vi "DAQ_2.vi"() -> ()   [LabVIEW 2021]
panel:
  in  "Fase":dbl(knob) scale=0.0..180.0
  in  "Frecuencia":dbl(knob) scale=0.0..30.0
  in  "Offset":dbl(knob) scale=-5.0..5.0
  in  "Amplitud":dbl(knob) scale=-5.0..5.0
  in  "Stop":bool
  out "Sine":dynamicdata(graph)
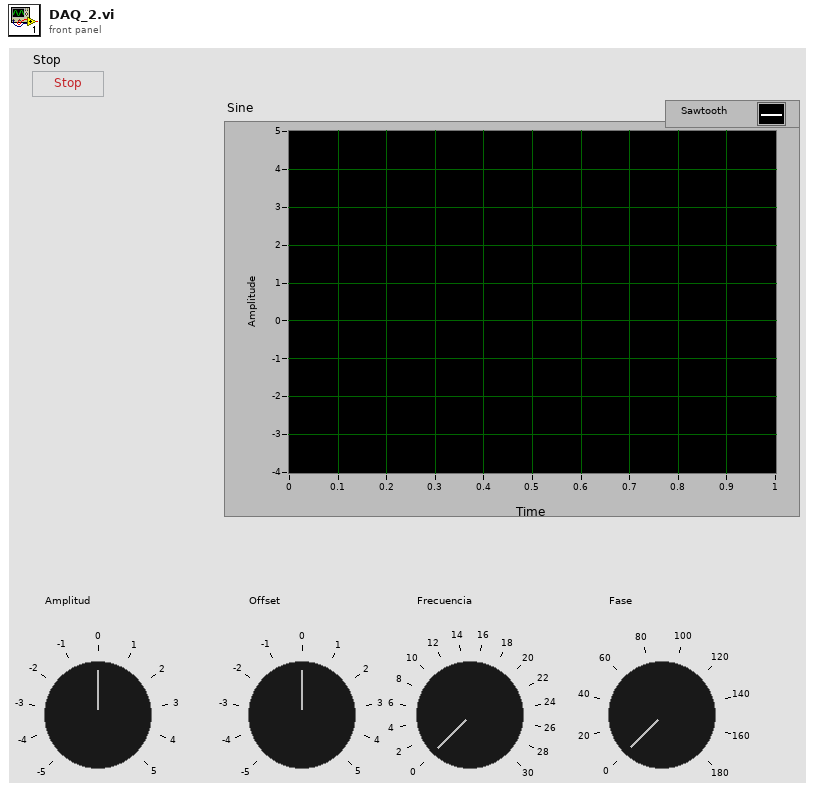
[diagram p1: front panel]
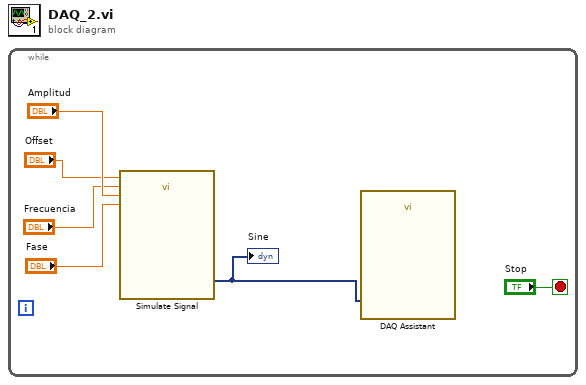
[diagram p0: block diagram]
diagram:
  n1 = while {
    stop <- "Stop" stop-if-true
    n2 = call "Simulate Signal"("Offset"="Offset", "Frequency"="Frecuencia", "Amplitude"="Amplitud", "Phase"="Fase") -> ("Sawtooth"=w5:dynamicdata)  [unwired: 10 in, 1 out]
    "Sine" <- w5
    n3 = call "DAQ Assistant"("data"=w5) -> ()  [unwired: 16 in, 3 out]
  }
